vi "Refresh.vi"(8 "error in (no error)":errorcluster, 11 "DeviceArrayPanel in":refnum<class "DeviceArrayPanel.lvclass">) -> (0 "error out":errorcluster, 3 "DeviceArrayPanel out":refnum<class "DeviceArrayPanel.lvclass">)   [LabVIEW 2020, in "PicoG-App.lvlib" / "DeviceArrayPanel.lvclass"]
uses:
  DeviceArrayPanel.lvclass
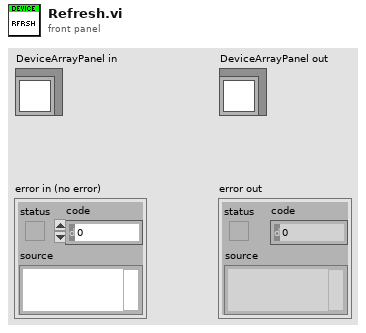
[diagram p1: front panel]
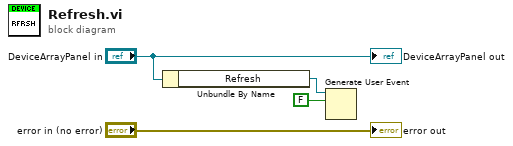
[diagram p0: block diagram]
diagram:
  n1 = Unbundle By Name("DeviceArrayPanel in") -> ("Refresh"=w2:refnum<user-event>)
  n2 = Generate User Event(user event=w2, event data cluster=FALSE ("event data")) -> ()  [unwired: 2 in, 2 out]
  "error out" <- "error in (no error)"
  "DeviceArrayPanel out" <- "DeviceArrayPanel in"
